vi "Plaintext to Morse Waveform.vi"(0 "Plaintext Array":string[](array[string]), 5 "Unit Speed (sec)":dbl=0.25 min=0.1 max=1.0 step=0.05, 7 "Character Gap":u8=3 min=2 max=6 step=1, 9 "Word Gap (Space)":u32=7 max=10 step=1, 11 "error in":errorcluster) -> (4 "waveform out":waveform(dbl), 15 "error out":errorcluster)   [LabVIEW 2026, in "Morse Sounder.lvlib"]
uses:
  Morse Sounder.lvlib
  <vilib>/Waveform/WDTOps.llb/WDT Append Waveforms DBL.vi
  <vilib>/measure/NI_MABase.lvlib
panel:
  out "Waveform Graph":waveform(dbl)(graph)
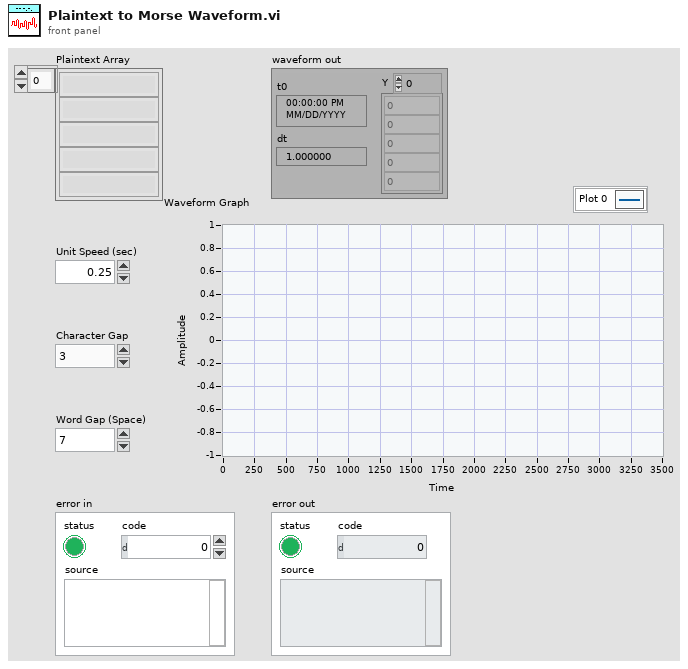
[diagram p1: front panel]
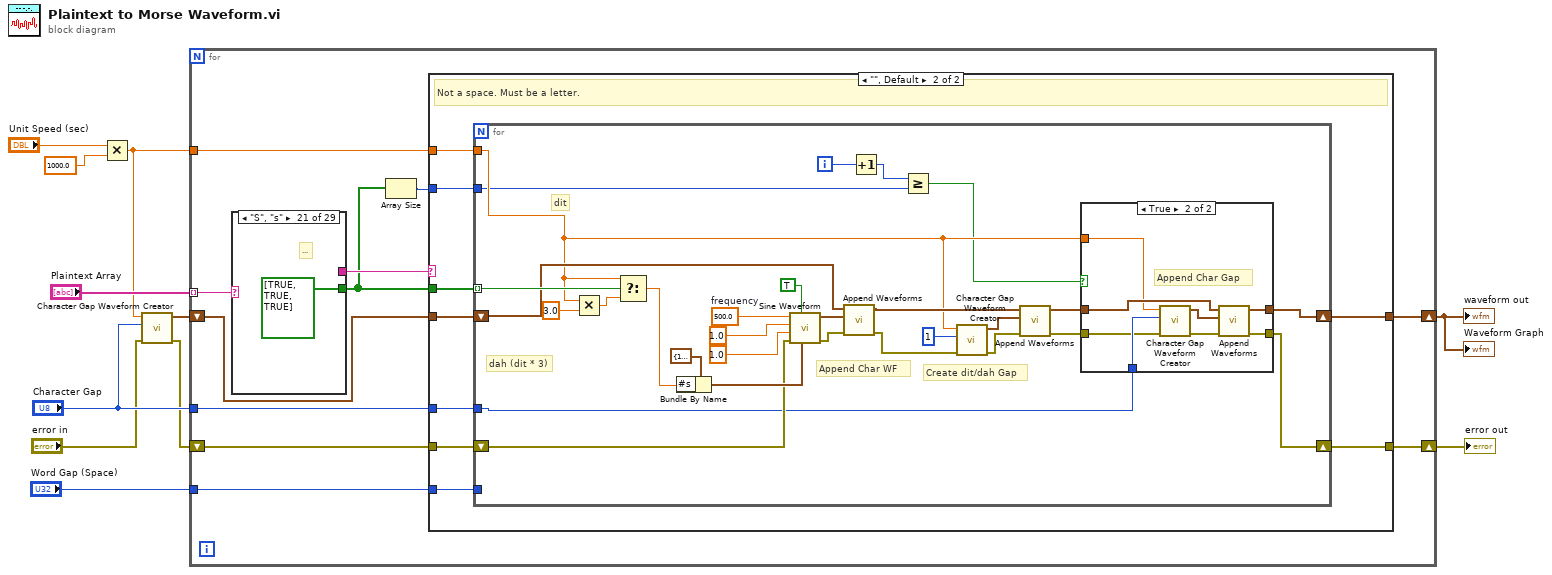
[diagram p0: block diagram]
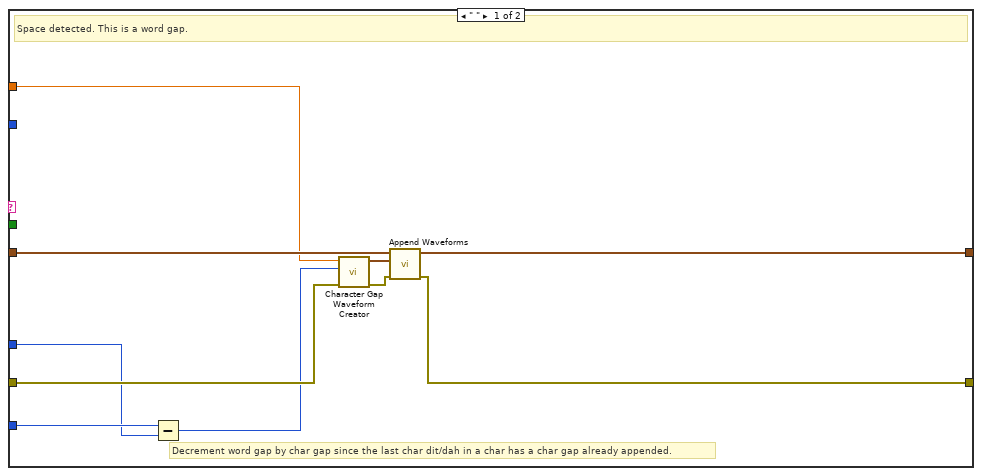
[diagram p2: hidden frame]
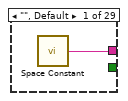
[diagram p4: hidden frame]
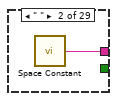
[diagram p5: hidden frame]
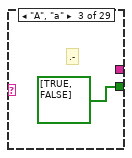
[diagram p6: hidden frame]
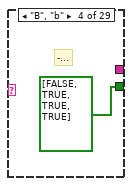
[diagram p7: hidden frame]
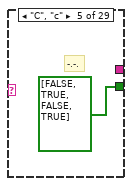
[diagram p8: hidden frame]
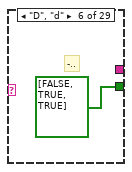
[diagram p9: hidden frame]
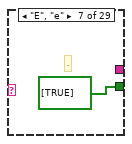
[diagram p10: hidden frame]
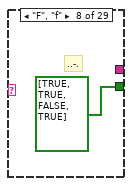
[diagram p11: hidden frame]
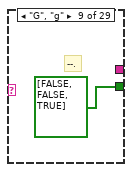
[diagram p12: hidden frame]
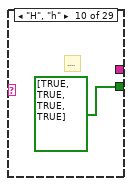
[diagram p13: hidden frame]
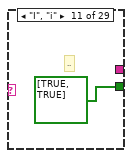
[diagram p14: hidden frame]
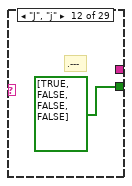
[diagram p15: hidden frame]
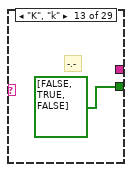
[diagram p16: hidden frame]
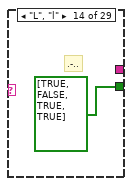
[diagram p17: hidden frame]
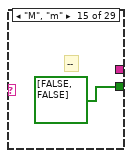
[diagram p18: hidden frame]
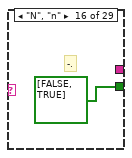
[diagram p19: hidden frame]
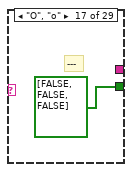
[diagram p20: hidden frame]
diagram:
  n1 = Multiply(x="Unit Speed (sec)", y=1000.0) -> (x*y=w4:dbl)
  n2 = call "Character Gap Waveform Creator.vi"("error in"="error in", "Character Gap"="Character Gap", "Numeric"=w4) -> ("error out"=w1:errorcluster, "waveform out"=w5:waveform(dbl))  [unwired: 7 in]
  n3 = for {
    tunnel: "Plaintext Array" -> [w22] mode=indexing
    tunnel: w4 -> [w21]
    tunnel: "Character Gap" -> [w20]
    tunnel: "Word Gap (Space)" -> [w18]
    shift-right: [w16] -> w7
    shift-left: w5 -> [w15]
    shift-right: [w14] -> w8
    shift-left: w1 -> [w19]
    n4 = case shown="\"S\", \"s\"" w22 {
      tunnel: [_ _ bool[] [TRUE, FALSE] bool[] [FALSE, TRUE, TRUE, TRUE] bool[] [FALSE, TRUE, FALSE, TRUE] bool[] [FALSE, TRUE, TRUE] bool[] [TRUE] bool[] [TRUE, TRUE, FALSE, TRUE] bool[] [FALSE, FALSE, TRUE] bool[] [TRUE, TRUE, TRUE, TRUE] bool[] [TRUE, TRUE] bool[] [TRUE, FALSE, FALSE, FALSE] bool[] [FALSE, TRUE, FALSE] bool[] [TRUE, FALSE, TRUE, TRUE] bool[] [FALSE, FALSE] bool[] [FALSE, TRUE] bool[] [FALSE, FALSE, FALSE] bool[] [TRUE, FALSE, FALSE, TRUE] bool[] [FALSE, FALSE, TRUE, FALSE] bool[] [TRUE, FALSE, TRUE] bool[] [TRUE, TRUE, TRUE] bool[] [FALSE] bool[] [TRUE, TRUE, FALSE] bool[] [TRUE, TRUE, TRUE, FALSE] bool[] [TRUE, FALSE, FALSE] bool[] [FALSE, TRUE, TRUE, FALSE] bool[] [FALSE, TRUE, FALSE, FALSE] bool[] [FALSE, FALSE, TRUE, TRUE] bool[] [TRUE, TRUE, FALSE, FALSE, TRUE, TRUE]] -> w13
      tunnel: [w81 w82 _ _ _ _ _ _ _ _ _ _ _ _ _ _ _ _ _ _ _ _ _ _ _ _ _ _ _] -> w17
      frame "", Default {
        n5 = call <vilib>:"Space Constant.vi"() -> ("String"=w81:string)
      }
      frame " " {
        n6 = call <vilib>:"Space Constant.vi"() -> ("String"=w82:string)
      }
      frame "A", "a" {
        # ".-"
      }
      frame "B", "b" {
        # "-..."
      }
      frame "C", "c" {
        # "-.-."
      }
      frame "D", "d" {
        # "-.."
      }
      frame "E", "e" {
        # "."
      }
      frame "F", "f" {
        # "..-."
      }
      frame "G", "g" {
        # "--."
      }
      frame "H", "h" {
        # "...."
      }
      frame "I", "i" {
        # ".."
      }
      frame "J", "j" {
        # ".---"
      }
      frame "K", "k" {
        # "-.-"
      }
      frame "L", "l" {
        # ".-.."
      }
      frame "M", "m" {
        # "--"
      }
      frame "N", "n" {
        # "-."
      }
      frame "O", "o" {
        # "---"
      }
      frame "P", "p" {
        # ".--."
      }
      frame "Q", "q" {
        # "--.-"
      }
      frame "R", "r" {
        # ".-."
      }
      frame "S", "s" {
        # "..."
      }
      frame "T", "t" {
        # "-"
      }
      frame "U", "u" {
        # "..-"
      }
      frame "V", "v" {
        # "...-"
      }
      frame "W", "w" {
        # ".--"
      }
      frame "X", "x" {
        # "-..-"
      }
      frame "Y", "y" {
        # "-.--"
      }
      frame "Z", "z" {
        # "--.."
      }
      frame "?" {
        # "..--.."
      }
    }
    n7 = Array Size(array=w13) -> (size(s)=w12:i32)
    n8 = case shown="\"\", Default" w17 {
      tunnel: w21 -> [w29 w41]
      tunnel: w20 -> [w23 w40]
      tunnel: w19 -> [w28 w39]
      tunnel: w18 -> [w24 w38]
      tunnel: w13 -> [_ w37]
      tunnel: [w31 w36] -> w16
      tunnel: w15 -> [w32 w35]
      tunnel: [w26 w34] -> w14
      tunnel: w12 -> [_ w33]
      frame " " {
        # "Decrement word gap by char gap since the last char dit/dah in a char has a char gap already appended."
        # "Space detected. This is a word gap."
        n9 = Subtract(x=w24, y=w23) -> (x-y=w25:u32)
        n10 = call "Character Gap Waveform Creator.vi"("error in"=w28, "Character Gap"=w25, "Numeric"=w29) -> ("error out"=w27:errorcluster, "waveform out"=w30:waveform(dbl))  [unwired: 7 in]
        n11 = call-poly <vilib>:"Append Waveforms.vi"("error in (no error)"=w27, "waveform B"=w30, "waveform A"=w32) -> ("error out"=w26:errorcluster, "waveform out"=w31:waveform(dbl))  [unwired: 7 in]
      }
      frame "", Default {
        # "Not a space. Must be a letter."
        n12 = for {
          tunnel: w37 -> [w64] mode=indexing
          tunnel: w41 -> [w46]
          tunnel: w40 -> [w51]
          shift-right: [w49] -> w36
          shift-left: w35 -> [w61]
          tunnel: w38 -> [_]
          shift-right: [w48] -> w34
          shift-left: w39 -> [w59]
          tunnel: w33 -> [w43]
          i -> [w45]
          w69 = 500.0  # frequency
          # "Create dit/dah Gap"
          # "Append Char WF"
          # "dah (dit * 3)"
          # "dit"
          n13 = Multiply(x=w46, y=3.0) -> (x*y=w63:dbl)
          n14 = Select(t=w46, s=w64, f=w63) -> (s? t:f=w57:dbl)
          n15 = Bundle By Name(cluster=cluster{"Fs":dbl, "#s":dbl} {"Fs"=1500.0, "#s"=1000.0} ("sampling info"), "#s"=w57) -> (w65:cluster{"Fs":dbl, "#s":dbl})
          n16 = call <vilib>:"Sine Waveform.vi"("sampling info"=w65, "reset signal"=TRUE, "error in (no error)"=w59, "phase"=1.0, "amplitude"=1.0, "frequency"=w69) -> ("error out"=w60:errorcluster, "signal out"=w62:waveform(dbl))  [unwired: 4 in]
          n17 = call-poly <vilib>:"Append Waveforms.vi"("error in (no error)"=w60, "waveform B"=w62, "waveform A"=w61) -> ("error out"=w55:errorcluster, "waveform out"=w56:waveform(dbl))  [unwired: 7 in]
          n18 = Increment(x=w45) -> (x+1=w42:i32)
          n19 = Greater Or Equal?(x=w42, y=w43) -> (x >= y?=w44:bool)
          n20 = call "Character Gap Waveform Creator.vi"("error in"=w55, "Character Gap"=u8 1, "Numeric"=w46) -> ("error out"=w53:errorcluster, "waveform out"=w54:waveform(dbl))  [unwired: 7 in]
          n21 = call-poly <vilib>:"Append Waveforms.vi"("error in (no error)"=w53, "waveform B"=w54, "waveform A"=w56) -> ("error out"=w50:errorcluster, "waveform out"=w47:waveform(dbl))  [unwired: 7 in]
          n22 = case shown="True" w44 {
            tunnel: w51 -> [_ w80]
            tunnel: w50 -> [w71 w79]
            tunnel: [w72 w77] -> w49
            tunnel: [w71 w76] -> w48
            tunnel: w47 -> [w72 w75]
            tunnel: w46 -> [_ w73]
            frame False {
            }
            frame True {
              # "Append Char Gap"
              n23 = call "Character Gap Waveform Creator.vi"("error in"=w79, "Character Gap"=w80, "Numeric"=w73) -> ("error out"=w78:errorcluster, "waveform out"=w74:waveform(dbl))  [unwired: 7 in]
              n24 = call-poly <vilib>:"Append Waveforms.vi"("error in (no error)"=w78, "waveform B"=w74, "waveform A"=w75) -> ("error out"=w76:errorcluster, "waveform out"=w77:waveform(dbl))  [unwired: 7 in]
            }
          }
        }
      }
    }
  }
  "waveform out" <- w7
  "error out" <- w8
  "Waveform Graph" <- w7
